vi "Get_Target_Type.vi"(8 "error in (no error)":errorcluster, 9 "install path":string, 10 "default install path":string, 11 "absFolder in":refnum<class "absFolder.lvclass">) -> (0 "error out":errorcluster, 1 "path for target type":T1=68 items=["Relative to default installation directory"=68, "Root directory on first partition"=70, "Relative to directory table key"=82, "Absolute path to file"=65], 2 "path for target":string, 3 "absFolder out":refnum<class "absFolder.lvclass">)   [LabVIEW 2020, in "absFolder.lvclass"]
uses:
  <vilib>/AppBuilder/IB_Classes/Destination/absFolder/absFolder.lvclass
  <vilib>/AppBuilder/IB_Classes/Destination/absFolder/absFolder.lvclass/absFolder.ctl
  AppLibs/distkit/MDF/NIMdf.llb/MDFBDPAddFilePathType.ctl
  AppLibs/distkit/MDF/NI_MDF.lvlib
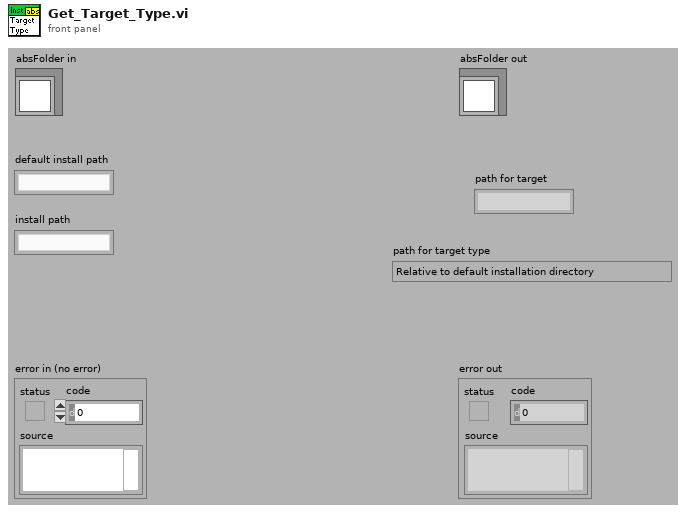
[diagram p1: front panel]
types:
  T1 = typedef "NI_MDF.lvlib/MDFBDPAddFilePathType.ctl" = i32
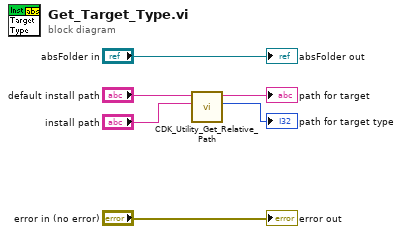
[diagram p0: block diagram]
diagram:
  n1 = call <resource>:"CDK_Utility_Get_Relative_Path.vi"("install path"="install path", "default install path"="default install path") -> ("path for target type"=→"path for target type":T1, "path for target"=→"path for target":string)  [unwired: 8 in]
  "error out" <- "error in (no error)"
  "absFolder out" <- "absFolder in"
